vi "Function Source Monitor.vi"(8 "error in (no error)":errorcluster, 9 "Curr Level Monitor (F: Off)":bool, 10 "Volt Level Monitor (F: Off)":bool, 11 "VISA resource name":refnum<visa-resource-name>) -> (0 "error out":errorcluster, 3 "VISA resource name out":refnum<visa-resource-name>)   [LabVIEW 2015, in "Agilent 428X Series.lvlib"]
doc: "This function sets the function source monitor VAC and IAC to the ON/OFF state."
uses:
  <instrlib>/Agilent 428X Series/Agilent 428X Series.lvlib
panel:
  # "On\nOff"
  # "On\nOff"
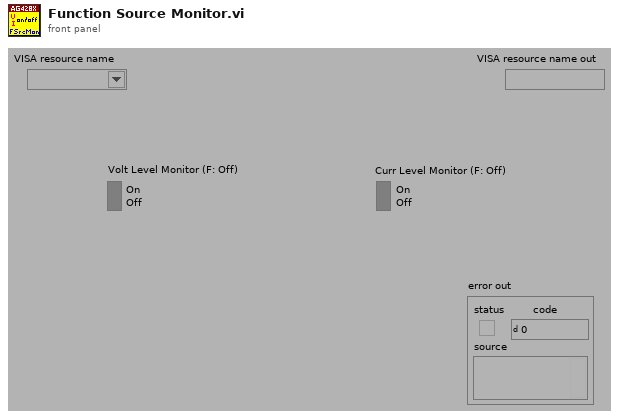
[diagram p1: front panel]
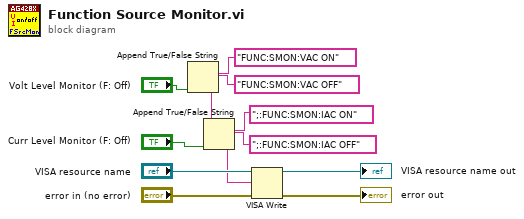
[diagram p0: block diagram]
diagram:
  n1 = Append True/False String(1:"Volt Level Monitor (F: Off)", 2:"FUNC:SMON:VAC OFF", 3:"FUNC:SMON:VAC ON") -> (0:w6:string)  [unwired: 1 in]
  n2 = Append True/False String(1:"Curr Level Monitor (F: Off)", 2:";:FUNC:SMON:IAC OFF", 3:";:FUNC:SMON:IAC ON", 4:w6) -> (0:w1:string)
  n3 = VISA Write(VISA resource name="VISA resource name", write buffer=w1, error in (no error)="error in (no error)") -> (VISA resource name out=→"VISA resource name out":refnum<visa-resource-name>, error out=→"error out":errorcluster)  [unwired: 1 out]
